vi "standard_uncertainty.vi"(2 "insieme":dbl[][](array[numeric])) -> (0 "Incertezza":dbl[](array[numeric]))   [LabVIEW 2021]
uses:
  <vilib>/Analysis/NI_AALBase.lvlib
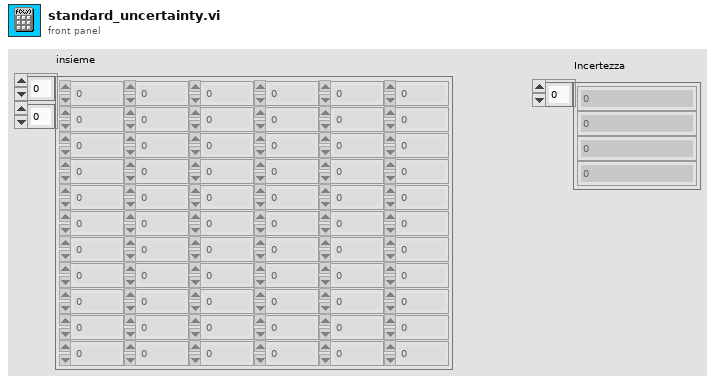
[diagram p1: front panel]
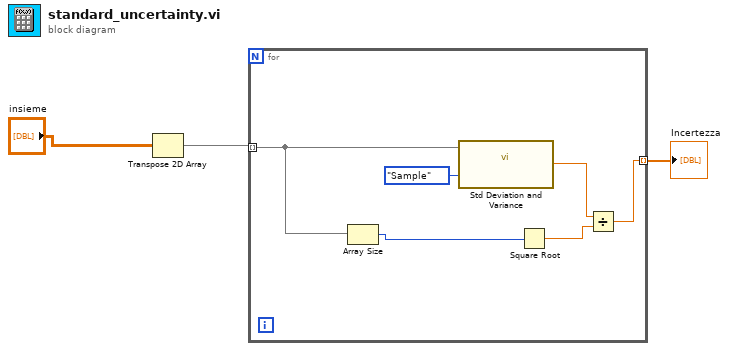
[diagram p0: block diagram]
diagram:
  n1 = Transpose 2D Array(2D array="insieme") -> (transposed array=w2:dbl[][])
  n2 = for {
    tunnel: [w6] -> w3 mode=indexing
    tunnel: w2 -> [w4] mode=indexing
    # "SALITA/DISCESA 1"
    n3 = Array Size(array=w4) -> (size(s)=w5:i32)
    n4 = call <vilib>:"Std Deviation and Variance.vi"("X"=w4, "Weighting (Sample)"=enum16{"Sample", "Population"}."Sample") -> ("standard deviation"=w7:dbl)  [unwired: 2 out]
    n5 = Square Root(x=w5) -> (sqrt(x)=w8:dbl)
    n6 = Divide(x=w7, y=w8) -> (x/y=w6:dbl)
  }
  "Incertezza" <- w3
